vi "Generate CSM Class mermaid(CSMH).vi"(8 "error in (no error)":errorcluster, 11 "CSM-Helper in":refnum<class "CSM-Helper.lvclass">) -> (0 "error out":errorcluster, 2 "resulting string":string, 3 "CSM-Helper out":refnum<class "CSM-Helper.lvclass">)   [LabVIEW 2020, in "CSM Mermaid Support.lvlib"]
uses:
  CSM Mermaid Support.lvlib
  <userlib>/_NEVSTOP/Communicable State Machine(CSM)/_csmHelper/CSM-Helper.lvclass
  <userlib>/_NEVSTOP/Communicable State Machine(CSM)/_csmHelper/CSM-Helper.lvclass/CSM-Helper.ctl
  <userlib>/_NEVSTOP/Communicable State Machine(CSM)/_csmHelper/Properties/Read VI Ref.vi
  <userlib>/_NEVSTOP/Communicable State Machine(CSM)/_csmHelper/API/Get All API Interface Info.vi
  <userlib>/_NEVSTOP/Communicable State Machine(CSM)/_csmHelper/API/Get Internal Data Info.vi
  <userlib>/_NEVSTOP/Communicable State Machine(CSM)/_csmHelper/API/Get All Status Interface Info.vi
  <userlib>/_NEVSTOP/Communicable State Machine(CSM)/Communicable State Machine.lvlib
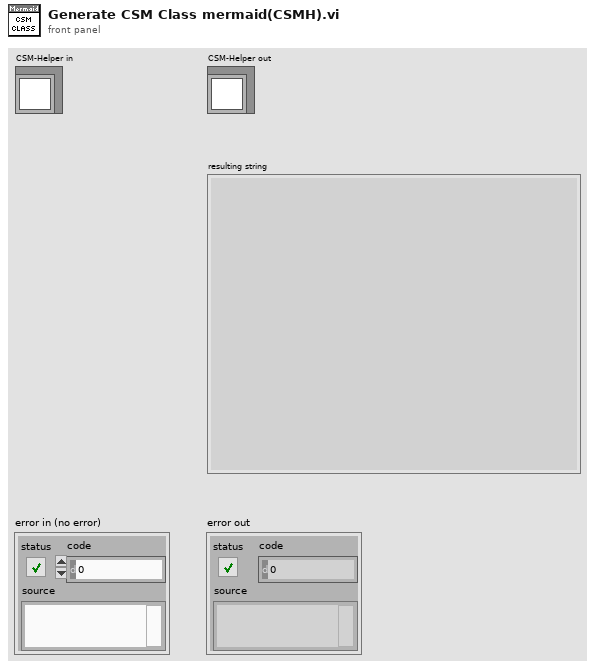
[diagram p1: front panel]
types:
  T1 = typedef "CSM-Helper.lvclass/Def-Argument Info.ctl" = cluster{"Type":string, "Name":string, "Variant":variant}
  T2 = typedef "CSM-Helper.lvclass/Def-Internal Data Info.ctl" = cluster{"Data":string, "prototype":variant}
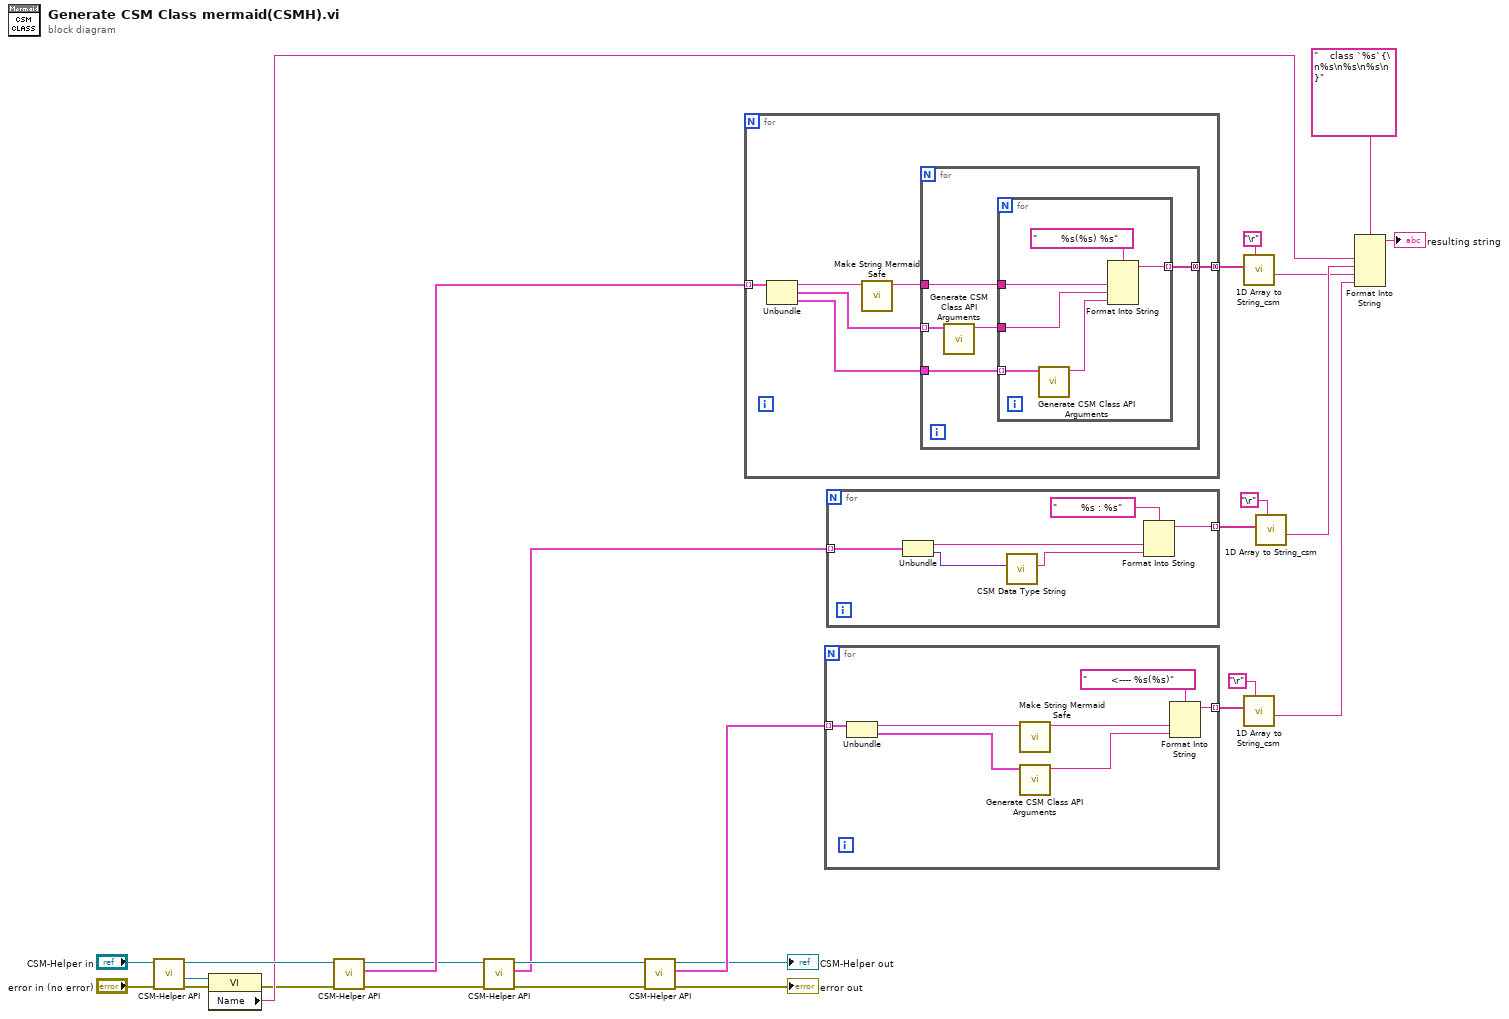
[diagram p0: block diagram]
diagram:
  n1 = call-poly <userlib>:"CSM-Helper API.vi"("error in (no error)"="error in (no error)", "CSM-Helper in"="CSM-Helper in") -> ("error out"=w3:errorcluster, "VI"=w1:refnum<vi>, "CSM-Helper out"=w27:refnum<class "CSM-Helper.lvclass">)  [unwired: 7 in]
  n2 = property on="Property Node" class="VI"(reference=w1, error in=w3) -> (error out=w2:errorcluster, "Name"=w9:string)  [unwired: 1 out]
  n3 = call-poly <userlib>:"CSM-Helper API.vi"("error in (no error)"=w2, "CSM-Helper in"=w27) -> ("error out"=w23:errorcluster, "Array"=w24:cluster{string, "Array":T1[], "Response":T1[]}[], "CSM-Helper out"=w22:refnum<class "CSM-Helper.lvclass">)  [unwired: 7 in]
  n4 = call-poly <userlib>:"CSM-Helper API.vi"("error in (no error)"=w23, "CSM-Helper in"=w22) -> ("error out"=w14:errorcluster, "Array"=w10:T2[], "CSM-Helper out"=w15:refnum<class "CSM-Helper.lvclass">)  [unwired: 7 in]
  n5 = call-poly <userlib>:"CSM-Helper API.vi"("error in (no error)"=w14, "CSM-Helper in"=w15) -> ("error out"=→"error out":errorcluster, "Array 3"=w20:cluster{string, "Argument":T1}[], "CSM-Helper out"=→"CSM-Helper out":refnum<class "CSM-Helper.lvclass">)  [unwired: 7 in]
  n6 = for {
    tunnel: [w33] -> w4 mode=concatenating
    tunnel: w24 -> [w31] mode=indexing
    n7 = Unbundle(w31) -> (w30:string, "Array"=w29:T1[], "Response"=w28:T1[])
    n8 = call "Make String Mermaid Safe.vi"("Source CSM"=w30) -> ("result string"=w32:string)  [unwired: 10 in]
    n9 = for {
      tunnel: [w38] -> w33 mode=concatenating
      tunnel: w32 -> [w37]
      tunnel: w29 -> [w36] mode=indexing
      tunnel: w28 -> [w34]
      n10 = call "Generate CSM Class API Arguments.vi"("Argument"=w36) -> ("String"=w35:string)  [unwired: 10 in]
      n11 = for {
        tunnel: w35 -> [w41]
        tunnel: w34 -> [w40] mode=indexing
        tunnel: w37 -> [w42]
        tunnel: [w43] -> w38 mode=indexing
        n12 = call "Generate CSM Class API Arguments.vi"("Argument"=w40) -> ("String"=w39:string)  [unwired: 10 in]
        n13 = Format Into String(format string="        %s(%s) %s", w42, w41, w39) -> (resulting string=w43:string)  [unwired: 2 in, 1 out]
      }
    }
  }
  n14 = for {
    tunnel: [w50] -> w19 mode=indexing
    tunnel: w20 -> [w48] mode=indexing
    n15 = Unbundle(w48) -> (w47:string, "Argument"=w46:T1)
    n16 = call "Make String Mermaid Safe.vi"("Source CSM"=w47) -> ("result string"=w49:string)  [unwired: 10 in]
    n17 = call "Generate CSM Class API Arguments.vi"("Argument"=w46) -> ("String"=w45:string)  [unwired: 10 in]
    n18 = Format Into String(format string="        <---- %s(%s)", w49, w45) -> (resulting string=w50:string)  [unwired: 2 in, 1 out]
  }
  n19 = for {
    tunnel: w10 -> [w56] mode=indexing
    tunnel: [w52] -> w12 mode=indexing
    n20 = Unbundle(w56) -> ("Data"=w55:string, "prototype"=w54:variant)
    n21 = call <userlib>:"CSM Data Type String.vi"("Data"=w54) -> ("Data Type String"=w53:string)  [unwired: 10 in]
    n22 = Format Into String(format string="        %s : %s", w55, w53) -> (resulting string=w52:string)  [unwired: 2 in, 1 out]
  }
  n23 = call <userlib>:"1D Array to String_csm.vi"("delimiter (Tab)"="\r" ("Carriage Return Constant"), "Array of Strings"=w4) -> ("delimited string"=w8:string)  [unwired: 9 in]
  n24 = call <userlib>:"1D Array to String_csm.vi"("delimiter (Tab)"="\r" ("Carriage Return Constant"), "Array of Strings"=w19) -> ("delimited string"=w21:string)  [unwired: 9 in]
  n25 = call <userlib>:"1D Array to String_csm.vi"("delimiter (Tab)"="\r" ("Carriage Return Constant"), "Array of Strings"=w12) -> ("delimited string"=w13:string)  [unwired: 9 in]
  n26 = Format Into String(format string="    class `%s`{\n%s\n%s\n%s\n    }", w9, w13, w8, w21) -> (resulting string=→"resulting string":string)  [unwired: 2 in, 1 out]
